vi "init daq state.vi"(0 "device":tag="Dev1", 11 "T cont wait time (ms)":i32=300) -> (4 "T cont out for global update":T1={"exec"={"T mode"=enum."Listening to exec", "log"=FALSE, "thermistor"=enum."solo"}, "T status"={"Temp"=0.0}, "utility"={"meas index"=0, "wait (ms)"=300, "therm volt"=0.0, "t T hist"=[]}} {"utility"."therm volt" format="%_6g"; "T status"."Temp" format="%_6g"}, 8 "DAQ state start out":T6 {"T cont"."utility"."therm volt" format="%_6g"; "T cont"."T status"."Temp" format="%_6g"})   [LabVIEW 2019]
doc: "Thus subvi initializes the temp daq state machine and the global variables for the thermistor experiment.\n\nPaul K Dixon\nP3600\nCSUSB Physics"
uses:
  typedefs/DAQ T state cluster.ctl
  typedefs/DAQ T state enum.ctl
  typedefs/temp cont cluster.ctl
  typedefs/temp exec cluster.ctl
  typedefs/temp mode enum.ctl
  typedefs/temp indicator.ctl
  typedefs/temp cont utility.ctl
panel:
  in  "T cont.T status":T4={"Temp"=25.0} {"Temp" format="%_6g"}
  in  "DAQ state start in":T6 {"T cont"."utility"."therm volt" format="%_6g"; "T cont"."T status"."Temp" format="%_6g"}
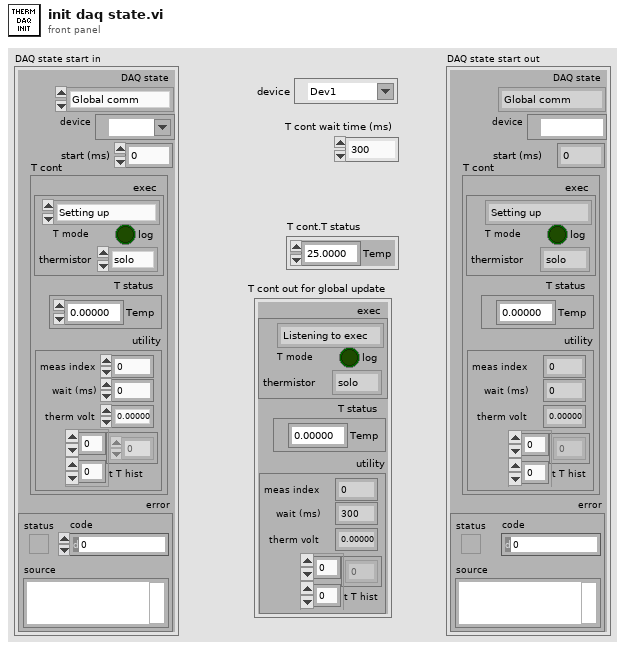
[diagram p1: front panel]
types:
  T1 = typedef "temp cont cluster.ctl" = cluster{"exec":T2, "T status":T4, "utility":T5}
  T2 = typedef "temp exec cluster.ctl" = cluster{"T mode":T3, "log":bool, "thermistor":enum16{"solo", "bug"}}
  T3 = typedef "temp mode enum.ctl" = enum16{"Setting up", "Listening to exec", "Exit"}
  T4 = typedef "temp indicator.ctl" = cluster{"Temp":dbl}
  T5 = typedef "temp cont utility.ctl" = cluster{"meas index":i32, "wait (ms)":i32, "therm volt":dbl, "t T hist":dbl[][]}
  T6 = typedef "DAQ T state cluster.ctl" = cluster{"DAQ state":T7, "device":tag, "start (ms)":i32, "error":errorcluster, "T cont":T1}
  T7 = typedef "DAQ T state enum.ctl" = enum16{"Global comm", "Meas T ", "Wait", "Exit"}
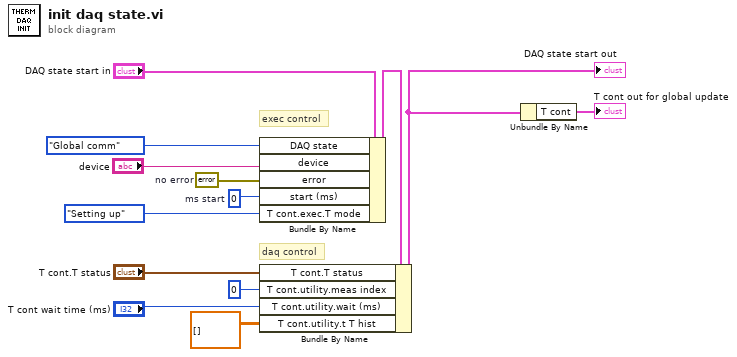
[diagram p0: block diagram]
diagram:
  w8 = u32 0  # ms start
  w11 = errorcluster {"status"=FALSE, "code"=0, "source"=""}  # no error
  # "daq control"
  # "exec control"
  n1 = Bundle By Name(cluster="DAQ state start in", "DAQ state"=DAQ_T_state_enum."Global comm", "device"="device", "error"=w11, "start (ms)"=w8, "T cont.exec.T mode"=temp_mode_enum."Setting up") -> (w10:T6)
  n2 = Bundle By Name(cluster=w10, "T cont.T status"="T cont.T status", "T cont.utility.meas index"=0 ("T cont.therm volt"), "T cont.utility.wait (ms)"="T cont wait time (ms)", "T cont.utility.t T hist"=dbl[][] [] ("T cont.T hist")) -> (w3:T6)
  "DAQ state start out" <- w3
  n3 = Unbundle By Name(w3) -> ("T cont"=→"T cont out for global update":T1)
